vi "u64 simple counter.vi"(11 "new fft cycle":bool) -> (3 "value":u64)   [LabVIEW 2021]
uses:
  <vilib>/rvi/FXPMathLib/basic elements/FxpAddSub/XNode/nifxpmath_AddSub.xnode
  <vilib>/rvi/FXPMathLib/sim/FxpSim.dll
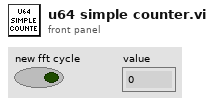
[diagram p1: front panel]
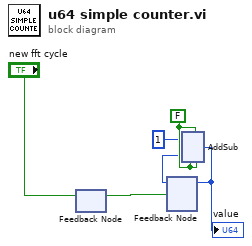
[diagram p0: block diagram]
diagram:
  w4 = FALSE ("use zero instead of x")
  n1 = feedback #1() -> (w5:bool)  [unwired: 1 in]
  n2 = feedback-in #1("new fft cycle") -> ()
  n3 = feedback #2() -> (w2:u64)  [unwired: 1 in]
  n4 = xnode "AddSub"("x"=u64 1, "y"=w2, "is sub?"=w4, "carry-in/inverted borrow-in"=w4, "use zero instead of x"=w4) -> ("s"=w3:u64)  [unwired: 1 out]
  "value" <- w3
  n5 = feedback-in #2(w3, w5) -> ()
